vi "Encoder.vi"() -> ()   [LabVIEW 2018]
doc: "I. Description:\nThis example demonstrates how to measure angular position using a quadrature encoder on a Counter Input Channel. The Decoding Type, Pulses Per Revolution, Z Index Enable, Z Index Phase, Z Index Value, and Sample Clock Source are all configurable. \n\nPosition is measured on the counter's default A, B, and Z input terminals (refer to section IV, I/O Connections Overview, below for more information).\n\nNote: For buffered position measurement, an external sample clock is necessary to signal when a sample should be inserted into the buffer. This is set by the Sample Clock Source control.\n\nII. Instructions for Running:\n1. Select the Physical Channel which corresponds to the counter you want to measure position on the DAQ device.\n2. Enter the Decoding Type, Pulses Per Revolution, Z Index Enable, Z Index Phase, Z Index Value to specify how you want the counter to measure position. Set the Sample Clock Source. \nNote: An external sample clock must be used. Counters do not have an internal sample clock available. You can use the Gen Dig Pulse Train-Continuous example to generate a pulse train on another counter and connect it to the Sample Clock Source you are using in this example.\n3. Set the Samples to Read control. This will determine how many samples are read each time the while loop iterates.\n\nIII. Block Diagram Steps:\n1. Create a Counter Input channel to Angular Encoder. The Decoding Type, Pulses Per Revolution, Z Index Enable, Z Index Phase, Z Index Value parameters are used to determine how the counter should measure position. \n2. Call the DAQmx Timing VI (Sample Clock) to configure the external sample clock timing parameters such as Sample Mode and Sample Clock Source. The Sample Clock Source determines when a sample will be inserted into the buffer. The 100kHz, 20MHz, and 80MHz timebases cannot be used as the Sample Clock Source. The Edge parameter can be used to determine when a sample is taken.\n3. Call the Start VI to arm the counter and begin measuring position. The counter will be preloaded with the Initial Angle.\n4. For continuous measurements, the counter will continually read all available data until the Stop button is pressed on the front panel.\n5. Call the Clear Task VI to clear the Task.\n6. Use the popup dialog box to display an error if any.\n\nIV. I/O Connections Overview: \nThe counter will measure position on the A, B, and Z Input Terminals of the counter specified in the Physical Channel I/O control.\n\nPosition measurement only works with TIO counters. \n\nFor more information on the default counter input and output terminals for your device, open the NI-DAQmx Help, and refer to Counter Signal Connections found under the Device Considerations book in the table of contents."
uses:
  <vilib>/DAQmx/read.llb/DAQmx Read (Counter 1D DBL 1Chan NSamp).vi
  <vilib>/DAQmx/create/channels.llb/DAQmx Create Channel (CI-Position-Angular Encoder).vi
  <vilib>/DAQmx/configure/timing.llb/DAQmx Timing (Sample Clock).vi
  <vilib>/DAQmx/miscellaneous.llb/DAQmx Fill In Error Info.vi
panel:
  out "Mean":dynamicdata(graph)
  out "Data":dbl[](graph)
  out "Waveform Graph":dynamicdata(graph)
  in  "Decoding Type":i32(ring)=10092 items=["X1"=10090, "X2"=10091, "X4"=10092, "Two Pulse Counting"=10313]
  in  "Pulses per Revolution":u32=1250
  in  "Counter(s)":tag="Dev1/ctr0" caption="Counter"
  in  "Rate":i32=100000 format="%.2e"
  in  "Sample Clock Source":tag="/Dev1/100kHzTimebase"
  in  "error in":errorcluster
  # "Channel Parameters"
  # "Timing Parameters"
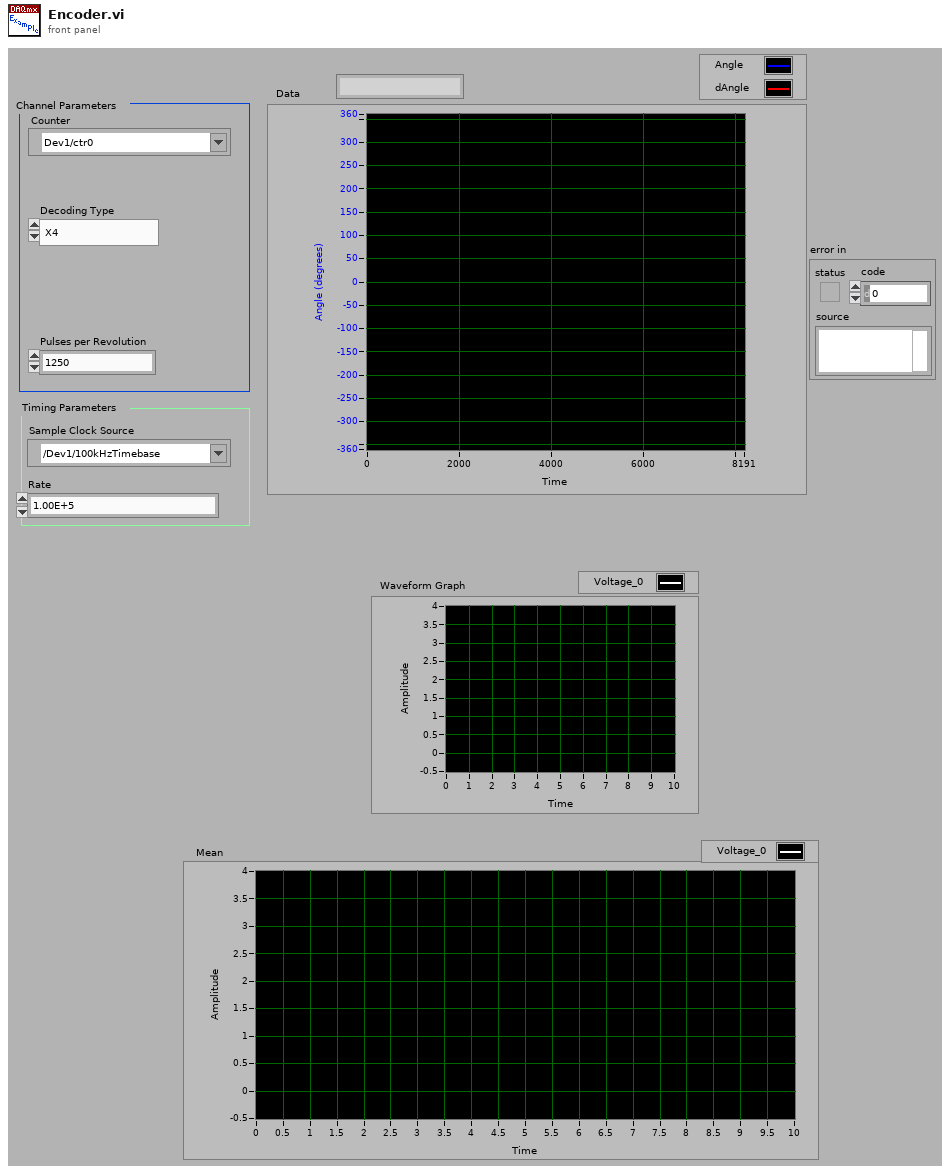
[diagram p1: front panel]
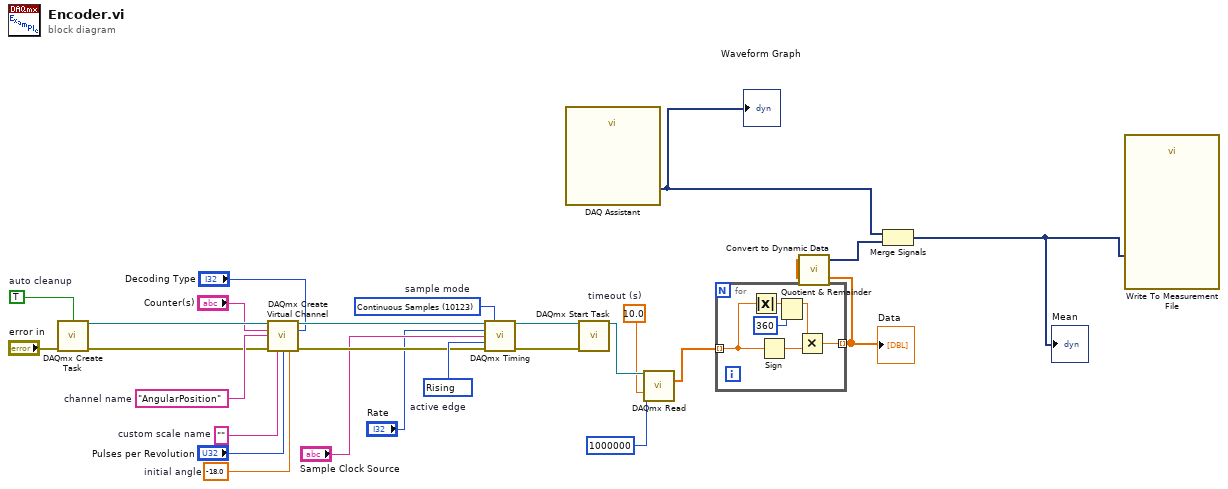
[diagram p0: block diagram]
diagram:
  w7 = 10.0  # timeout (s)
  w25 = 10123 items=["Finite Samples"=10178, "Continuous Samples"=10123, "Hardware Timed Single Point"=12522]  # sample mode
  w24 = 10280 items=["Rising"=10280, "Falling"=10171]  # active edge
  w23 = -18.0  # initial angle
  w22 = ""  # custom scale name
  w21 = "AngularPosition"  # channel name
  w18 = TRUE  # auto cleanup
  n1 = call <vilib>:"DAQmx Create Task.vi"("auto cleanup"=w18, "error in"="error in") -> ("task out"=w19:refnum<k21>, "error out"=w17:errorcluster)  [unwired: 12 in]
  n2 = call-poly <vilib>:"DAQmx Create Virtual Channel.vi"("task in"=w19, "counter"="Counter(s)", "decoding type"="Decoding Type", "name to assign"=w21, "error in"=w17, "custom scale name"=w22, "pulses per revolution"="Pulses per Revolution", "initial angle"=w23) -> ("task out"=w13:refnum<k21>, "error out"=w20:errorcluster)  [unwired: 6 in]
  n3 = call-poly <vilib>:"DAQmx Timing.vi"("task/channels in"=w13, "sample mode"=w25, "rate"="Rate", "source"="Sample Clock Source", "active edge"=w24, "error in"=w20) -> ("task out"=w14:refnum<k21>, "error out"=w15:errorcluster)  [unwired: 8 in]
  n4 = call "DAQ Assistant"() -> ("data"=w3:dynamicdata)  [unwired: 17 in, 2 out]
  "Waveform Graph" <- w3
  n5 = call <vilib>:"DAQmx Start Task.vi"("task/channels in"=w14, "error in"=w15) -> ("task out"=w26:refnum<k21>)  [unwired: 12 in, 1 out]
  n6 = call-poly <vilib>:"DAQmx Read.vi"("task/channels in"=w26, "number of samples per channel"=1000000, "timeout"=w7) -> ("data"=w6:dbl[])  [unwired: 10 in, 2 out]
  n7 = for {
    tunnel: w6 -> [w32] mode=indexing
    tunnel: [w27] -> w5 mode=indexing
    n8 = Absolute Value(x=w32) -> (abs(x)=w30:dbl)
    n9 = Sign(1:w32) -> (0:w28:dbl)
    n10 = Quotient & Remainder(x=w30, y=360) -> (x-y*floor(x/y)=w29:dbl)  [unwired: 1 out]
    n11 = Multiply(x=w29, y=w28) -> (x*y=w27:dbl)
  }
  "Data" <- w5
  n12 = call "Convert to Dynamic Data"("Array"=w5) -> ("Dynamic Data Type"=w2:dynamicdata)  [unwired: 3 in]
  n13 = Merge Signals(w3, w2) -> (w1:dynamicdata)
  "Mean" <- w1
  n14 = call "Write To Measurement File"("Signals"=w1) -> ()  [unwired: 16 in, 3 out]
